vi "celsiusandfahrenheit2.vi"() -> ()   [LabVIEW 2018]
panel:
  in  "?":bool
  out "?":string
  in  "Celsius or Fahrenheit":bool
  out "?":dbl
  out "?":dbl(slide) scale=-30.0..125.0
  out "Celsius":dbl
  in  "Slide":dbl(slide) scale=-30.0..50.0
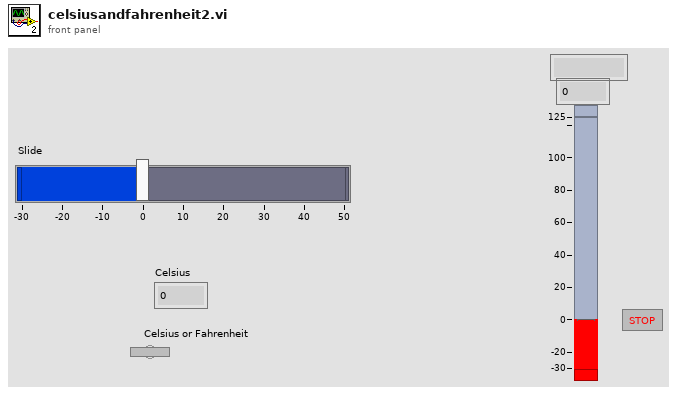
[diagram p1: front panel]
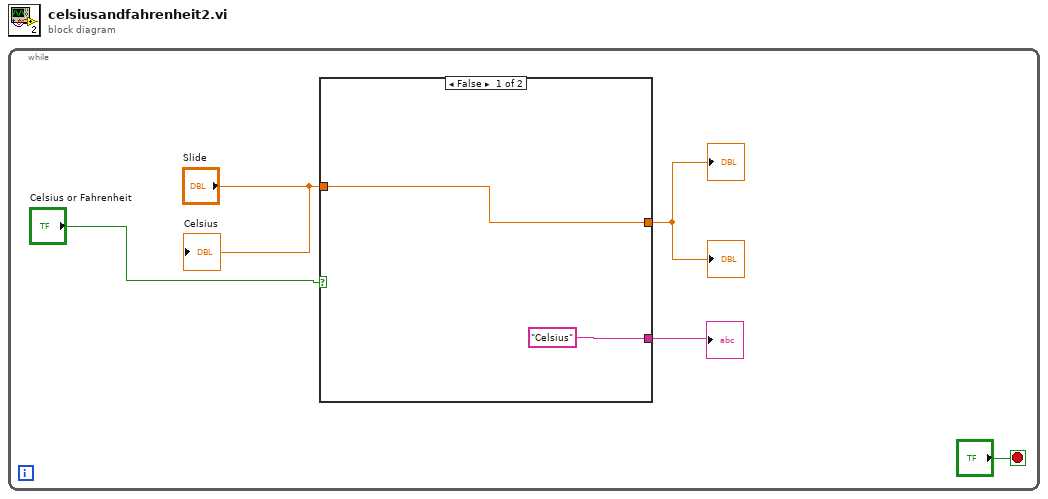
[diagram p0: block diagram]
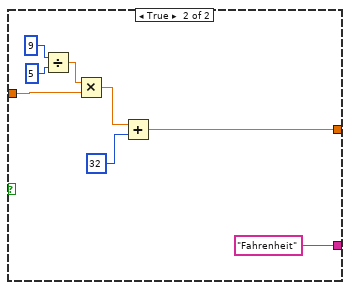
[diagram p2: hidden frame]
diagram:
  n1 = while {
    stop <- "?" stop-if-true
    n2 = case shown="False" "Celsius or Fahrenheit" {
      tunnel: "Slide" -> [w7 w10]
      tunnel: [w7 w9] -> w3
      tunnel: ["Celsius" "Fahrenheit"] -> w2
      frame False {
      }
      frame True {
        n3 = Divide(x=9, y=5) -> (x/y=w15:dbl)
        n4 = Multiply(x=w15, y=w10) -> (x*y=w12:dbl)
        n5 = Add(x=w12, y=32) -> (x+y=w9:dbl)
      }
    }
    "?" <- w3
    "?" <- w3
    "?" <- w2
    "Celsius" <- "Slide"
  }
